vi "Configure Channels.vi"(8 "error in":errorcluster, 11 "AO DAQmx DC CFG in":refnum<class "AO DAQmx DC CFG.lvclass">) -> (0 "error out":errorcluster, 3 "AO DAQmx DC CFG out":refnum<class "AO DAQmx DC CFG.lvclass">)   [LabVIEW 2023, in "AO DAQmx DC CFG.lvclass"]
uses:
  AO DAQmx DC CFG.lvclass
  AO DAQmx DC CFG.lvclass/AO DAQmx DC CFG.ctl
  DAQmx Base CFG/DAQmx Base CFG.lvclass/DAQmx Base CFG.ctl
  Configurations/CFG Base/CFG Base.lvclass/CFG Base.ctl
  2706bce0-41ed-4706-90a9-e9d573054dd0.vi
  <vilib>/JDP Science/JSONtext/Find Item.vi
  <vilib>/JDP Science/JSONtext/Next JSON Value.vi
  <vilib>/JDP Science/JSONtext/String Subset.vi
  <vilib>/JDP Science/JSONtext/Parsing/Advance past next JSON Value (inlined COPY).vi
  <vilib>/JDP Science/JSONtext/Parsing/Advance past whitespace.vi
  <vilib>/JDP Science/JSONtext/Parsing/Advance past String.vi
  <vilib>/JDP Science/JSONtext/Parsing/Advance past Number.vi
  <vilib>/JDP Science/JSONtext/Parsing/Advance past Line Ending.vi
  <vilib>/JDP Science/JSONtext/Parsing/Parse Full Path or Item Name.vi
  <vilib>/JDP Science/JSONtext/Parsing/Advance past Array.vi
  <vilib>/JDP Science/JSONtext/Parsing/Advance past Object.vi
  <vilib>/JDP Science/JSONtext/support/Error Cluster From Code.vi
  <vilib>/JDP Science/JSONtext/Offset/Find Item Locations by Path.vi
  <vilib>/JDP Science/JSONtext/JSON text to Variant.vi
  <vilib>/Utility/error.llb/Error Cluster From Error Code.vi
  <vilib>/DAQmx/create/channels.llb/DAQmx Create Channel (AO-Voltage-Basic).vi
  <vilib>/JDP Science/JSONtext/LVClass Serializer/JSONtext LVClass Serializer.lvclass
  <vilib>/ErrorRing/Error Ring.xnode
  Buffers/BufferWrites1SamDBL/BufferWrites1SamDBL.lvclass
  DAQmx Base CFG/DAQmx Base CFG.lvclass
  Configurations/CFG JSON/CFG JSON.lvclass
  Configurations/CFG Base/CFG Base.lvclass
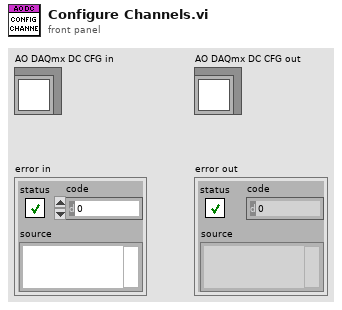
[diagram p1: front panel]
types:
  T1 = cluster{"Name":string, "Enabled":bool, "Maximum Value":dbl, "Minimum Value":dbl, "Output Terminal CFG":string, "Units":string, "Level":dbl}[]
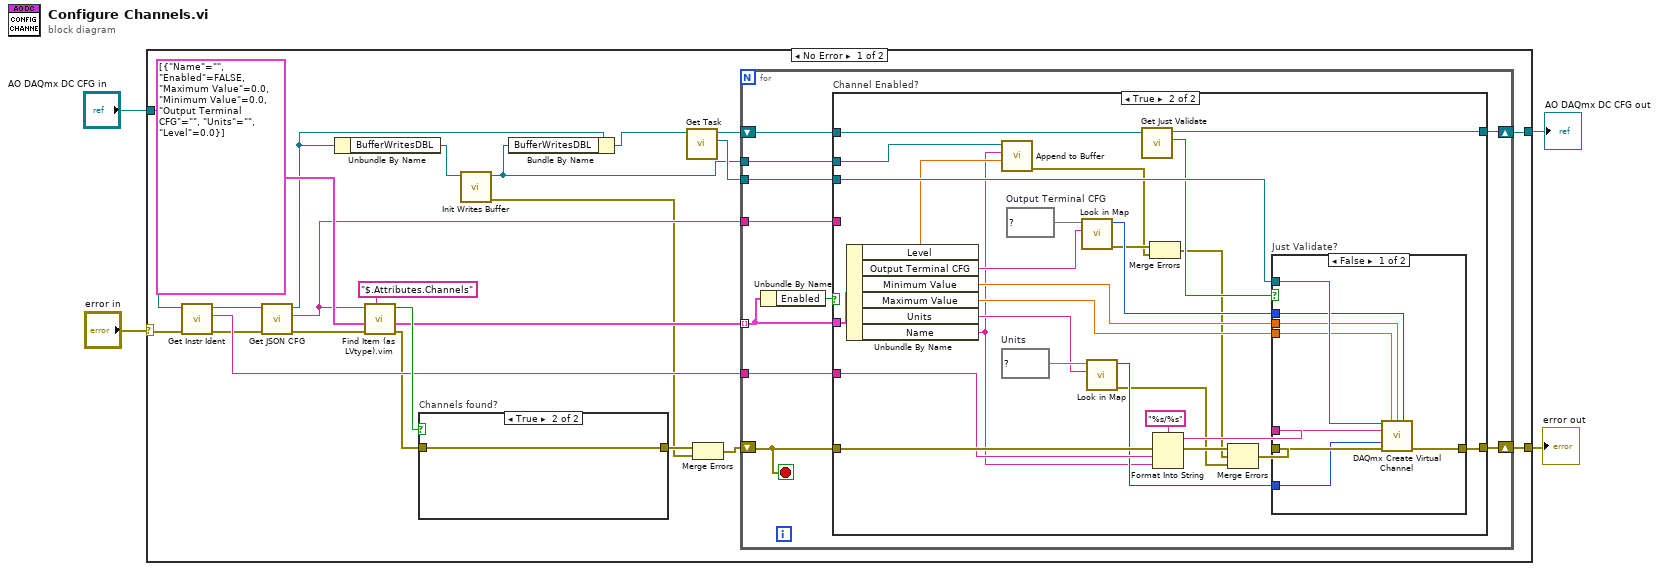
[diagram p0: block diagram]
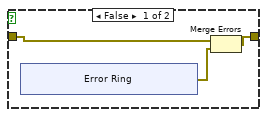
[diagram p2: hidden frame]
diagram:
  n1 = case shown="No Error" "error in" {
    selector: "error in" -> [w20 w84]
    tunnel: "AO DAQmx DC CFG in" -> [w16 w85]
    tunnel: [w21 w84] -> w2
    tunnel: [w15 w85] -> w1
    frame No Error {
      n2 = call-dynamic "Get Instr Ident.vi"("error in"=w20, "CFG JSON in"=w16) -> ("error out"=w11:errorcluster, "Instr Ident"=w22:string, "CFG JSON out"=w23:refnum<class "AO DAQmx DC CFG.lvclass">)  [unwired: 7 in]
      n3 = call "Get JSON CFG.vi"("CFG JSON in"=w23) -> ("<JSON> CFG"=w19:string, "CFG JSON out"=w9:refnum<class "AO DAQmx DC CFG.lvclass">)  [unwired: 9 in]
      n4 = Unbundle By Name(w9) -> ("BufferWritesDBL"=w10:refnum<class "BufferWrites1SamDBL.lvclass">)
      n5 = call "Find Item (as LVtype).vim"("$Path or Item Name"="$.Attributes.Channels", "error in (no error)"=w11, "Data Type and Default Value"=T1 [{"Name"="", "Enabled"=FALSE, "Maximum Value"=0.0, "Minimum Value"=0.0, "Output Terminal CFG"="", "Units"="", "Level"=0.0}], "JSON"=w19) -> ("error out"=w12:errorcluster, "Data"=w17:T1, "Found"=w25:bool)  [unwired: 4 in, 1 out]
      n6 = case "Channels found?" shown="True" w25 {
        tunnel: w12 -> [w29 w35]
        tunnel: [w27 w35] -> w13
        frame False {
          n7 = xnode "Error Ring"() -> ("error out"=w28:errorcluster)
          n8 = Merge Errors(w29, w28) -> (w27:errorcluster)
        }
        frame True {
        }
      }
      n9 = call-dynamic "Init Writes Buffer.vi"("BufferWrites1SamDBL in"=w10) -> ("error out"=w6:errorcluster, "BufferWrites1SamDBL out"=w5:refnum<class "BufferWrites1SamDBL.lvclass">)  [unwired: 9 in]
      n10 = Bundle By Name(cluster=w9, "BufferWritesDBL"=w5) -> (w8:refnum<class "AO DAQmx DC CFG.lvclass">)
      n11 = call "Get Task.vi"("DAQmx Base CFG in"=w8) -> ("Task"=w18:refnum<k21>, "DAQmx Base CFG out"=w14:refnum<class "AO DAQmx DC CFG.lvclass">)  [unwired: 9 in]
      n12 = Merge Errors(w13, w6) -> (w7:errorcluster)
      n13 = for {
        tunnel: w17 -> [w42] mode=indexing
        shift-right: [w45] -> w21
        shift-left: w7 -> [w44]
        tunnel: w22 -> [w43]
        tunnel: w19 -> [w41]
        tunnel: w18 -> [w40]
        shift-right: [w39] -> w15
        shift-left: w14 -> [w38]
        tunnel: w5 -> [w36]
        stop <- w44 stop-if-true
        n14 = Unbundle By Name(w42) -> ("Enabled"=w37:bool)
        n15 = case "Channel Enabled?" shown="True" w37 {
          tunnel: [w47 w52] -> w45
          tunnel: w44 -> [w47 w71]
          tunnel: w43 -> [_ w70]
          tunnel: w42 -> [_ w74]
          tunnel: [w46 w63] -> w39
          tunnel: w41 -> [_ _]
          tunnel: w40 -> [_ w73]
          tunnel: w38 -> [w46 w55]
          tunnel: w36 -> [_ w56]
          frame False {
          }
          frame True {
            w59 = map{string, i32} {"From Custom Scale"=10065, "Volts"=10348}  # Units
            w66 = map{string, i32} {"Default"=-1, "Differential"=10106, "Pseudodifferential"=12529, "RSE"=10083}  # Output Terminal CFG
            n16 = Unbundle By Name(w74) -> ("Level"=w51:dbl, "Output Terminal CFG"=w65:string, "Minimum Value"=w61:dbl, "Maximum Value"=w60:dbl, "Units"=w58:string, "Name"=w50:string)
            n17 = call-dynamic "Append to Buffer.vi"("Level"=w51, "Ident"=w50, "BufferWrites1SamDBL in"=w56) -> ("error out"=w48:errorcluster)  [unwired: 7 in, 1 out]
            n18 = call "Look in Map.vi"("Key"=w65, "Map"=w66) -> ("error out"=w54:errorcluster, "Value"=w64:i32)  [unwired: 8 in]
            n19 = call "Look in Map.vi"("Key"=w58, "Map"=w59) -> ("error out"=w53:errorcluster, "Value"=w57:i32)  [unwired: 8 in]
            n20 = call "Get Just Validate.vi"("CFG Base in"=w55) -> ("Just Validate"=w62:bool, "CFG Base out"=w63:refnum<class "AO DAQmx DC CFG.lvclass">)  [unwired: 9 in]
            n21 = Merge Errors(w54, w48) -> (w49:errorcluster)
            n22 = Format Into String(format string="%s/%s", error in=w71, w70, w50) -> (resulting string=w68:string, error out=w69:errorcluster)  [unwired: 1 in]
            n23 = Merge Errors(w69, w49, w53) -> (w67:errorcluster)
            n24 = case "Just Validate?" shown="False" w62 {
              tunnel: w67 -> [w82 w83]
              tunnel: w68 -> [w79 _]
              tunnel: w73 -> [w81 _]
              tunnel: [w80 w83] -> w52
              tunnel: w64 -> [w78 _]
              tunnel: w61 -> [w77 _]
              tunnel: w60 -> [w76 _]
              tunnel: w57 -> [w75 _]
              frame False {
                n25 = call-poly <vilib>:"DAQmx Create Virtual Channel.vi"("task in"=w81, "maximum value"=w76, "minimum value"=w77, "output terminal configuration"=w78, "physical channels"=w79, "units"=w75, "error in"=w82) -> ("error out"=w80:errorcluster)  [unwired: 7 in, 1 out]
              }
              frame True {
              }
            }
          }
        }
      }
    }
    frame Error {
    }
  }
  "error out" <- w2
  "AO DAQmx DC CFG out" <- w1
